vi "IMAQdx Discover Ethernet Cameras.vi"(7 "Timeout (1000 ms)":u32=1000, 8 "error in":errorcluster, 11 "Address (Broadcast)":string="255.255.255.255") -> (0 "error out":errorcluster)   [LabVIEW 2020, in "NI_Vision_Acquisition_Software.lvlib"]
doc: "Initiates a round of Ethernet camera discovery. Use this VI to find Ethernet cameras on the network with a remote subnet. This VI will be blocked and will return after the specified timeout. The address specifies the destination address for the discovery command. The default address is 255.255.255.255. Call this VI before calling IMAQdx Enumerate Cameras VI or IMAQdx Open Camera VI."
uses:
  NI_Vision_Acquisition_Software.lvlib
  niimaqdx.dll
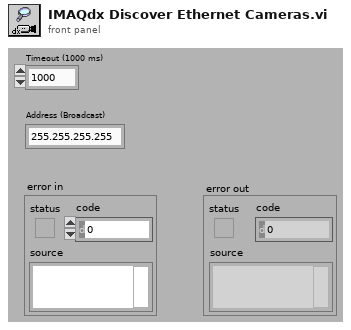
[diagram p1: front panel]
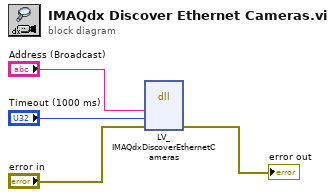
[diagram p0: block diagram]
diagram:
  n1 = dll-call lib="niimaqdx.dll" fn="LV_IMAQdxDiscoverEthernetCameras"("address"="Address (Broadcast)", "timeout"="Timeout (1000 ms)", "error in"="error in") -> ("error in"=→"error out":errorcluster)  [unwired: 6 in, 2 out]
